vi "GetSetTempDir.vi"(3 "Path":refnum<vi>) -> ()   [LabVIEW 2009]
panel:
  out "rebinning after":dbl
  out "rebinning before":dbl
  in  "rebinning":dbl
  in  "false color palette":T1 {"Numeric 12" format="%.0x"; "Numeric 11" format="%.0x"; "Numeric 10" format="%.0x"; "Numeric 9" format="%.0x"; "Numeric 8" format="%.0x"; "Numeric 7" format="%.0x"; "Numeric 6" format="%.0x"; "Numeric 5" format="%.0x"; "Numeric 4" format="%.0x"; "Numeric 3" format="%.0x"; "Numeric 2" format="%.0x"; "Numeric" format="%.0x"}
  out "colors":u32[](array[colorbox])
  in  "ADC-Resolution":u16(ring) items=["8bit", "12bit", "4bit"]
  in  "raw data screen":bool
  in  "Fileformat":enum16{"Herty", "Ken", "SPC130", "HydraHarp"}(ring)
  in  "stop":bool
  in  "Path for .tmp-files":path
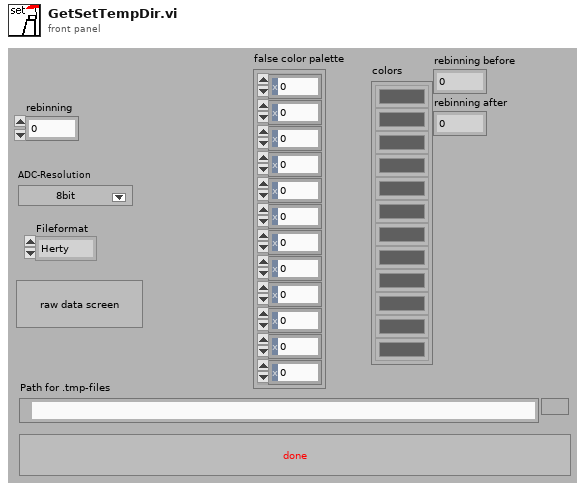
[diagram p1: front panel]
types:
  T1 = cluster{"Numeric":u32, "Numeric 2":u32, "Numeric 3":u32, "Numeric 4":u32, "Numeric 5":u32, "Numeric 6":u32, "Numeric 7":u32, "Numeric 8":u32, "Numeric 9":u32, "Numeric 10":u32, "Numeric 11":u32, "Numeric 12":u32}
  T2 = typedef "Settings.ctl" = cluster{"threshold":cluster{"max":u32, "min":u32}, "RGB or false color":bool, "16bit":bool, "log/lin axis":u16, "spotsize button":bool, "Pixelsize":u16, "autoscale x":bool, "autoscale y":bool, "correlation":bool, "ADC-Resolution":i32, "F2-lifetime":cluster{"display tau":bool, "display F2":bool, "Palette Number lifetime":enum32{"Gray", "Binary", "Gradient", "Rainbow", "Temperature"}, "Palette Number F2":enum32{"Gray", "Binary", "Gradient", "Rainbow", "Temperature"}, "max tau-Value":dbl, "min tau-Value":dbl, "max F2-Value":dbl, "min F2-Value":dbl}, "TAC-Window 1":u16, "TAC-Window 2":u16, "false color palette":cluster{"1":u32, "2":u32, "3":u32, "4":u32, "5":u32, "6":u32, "7":u32, "8":u32, "8 2":u32, "8 3":u32, "8 4":u32, "8 5":u32}, "rebinning":dbl}
  T3 = cluster{"1":u32, "2":u32, "3":u32, "4":u32, "5":u32, "6":u32, "7":u32, "8":u32, "8 2":u32, "8 3":u32, "8 4":u32, "8 5":u32}
  T4 = typedef "FIFOSettings_BH.ctt" = cluster{"Measurement":cluster{"Binning (ms)":sgl, "External Trigger Condition":u16, "Stop Condition:":u16, "Stop Count":dbl, "Buffer Size (Photons)":u16, "No of Channels":u16, "Ext Latch Delay":i16}, "ADC":cluster{"Module":u16, "ADC Resolution":i32, "Dither Range":i16, "Count Increment":i16, "Macro Time Clock":i16}, "SYNC":cluster{"SYNC ZC Level (mV)":sgl, "SYNC Freq Divider":i16, "SYNC Holdoff (ns)":sgl, "SYNC Threshold (mV)":sgl}, "TAC":cluster{"TAC Range (ns)":sgl, "TAC Gain":i16, "TAC Offset (%)":sgl, "TAC Limit Low (%)":sgl, "TAC Limit High (%)":sgl}, "CFD":cluster{"CFD Limit Low (mV)":sgl, "CFD Limit High (mV)":sgl, "CFD ZC Level (mV)":sgl, "CFD Holdoff (ns)":sgl}}
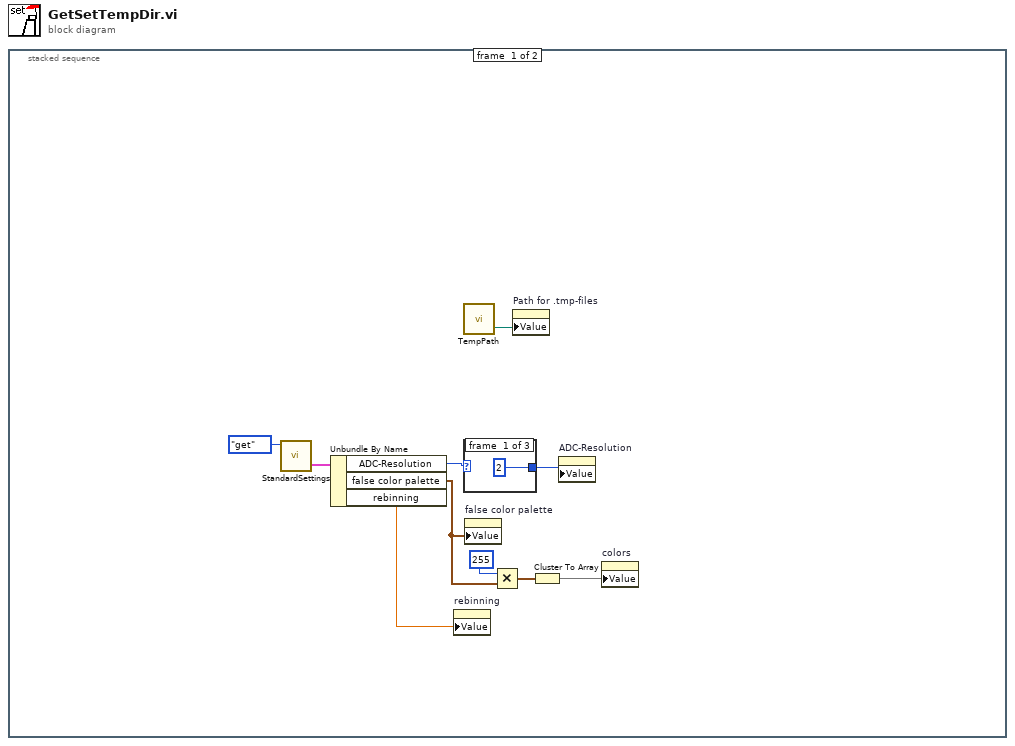
[diagram p0: block diagram]
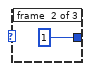
[diagram p2: hidden frame]
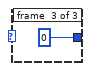
[diagram p3: hidden frame]
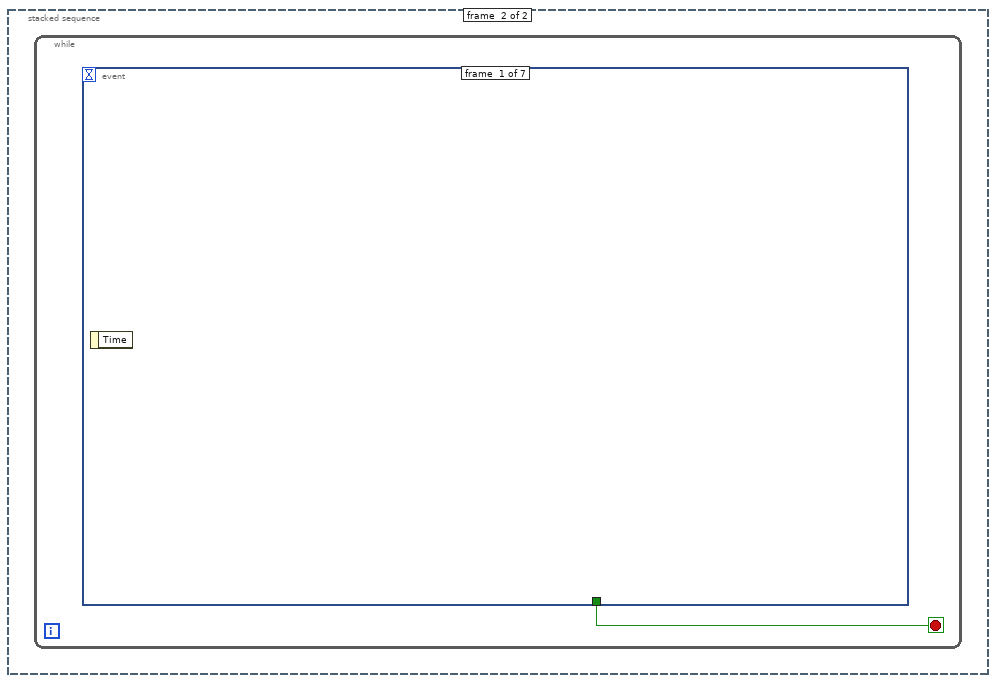
[diagram p4: hidden frame]
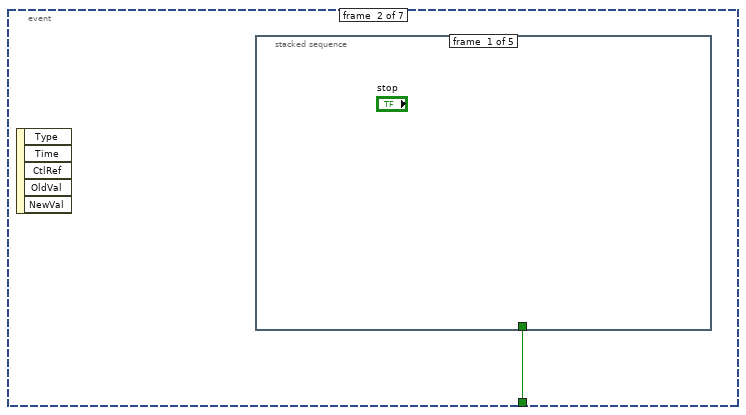
[diagram p5: hidden frame]
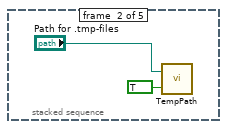
[diagram p6: hidden frame]
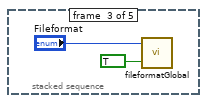
[diagram p7: hidden frame]
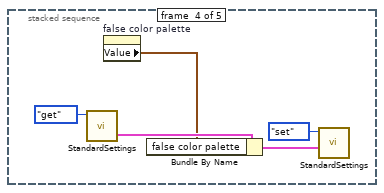
[diagram p8: hidden frame]
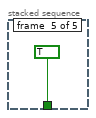
[diagram p9: hidden frame]
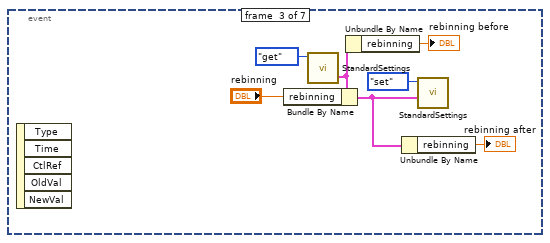
[diagram p10: hidden frame]
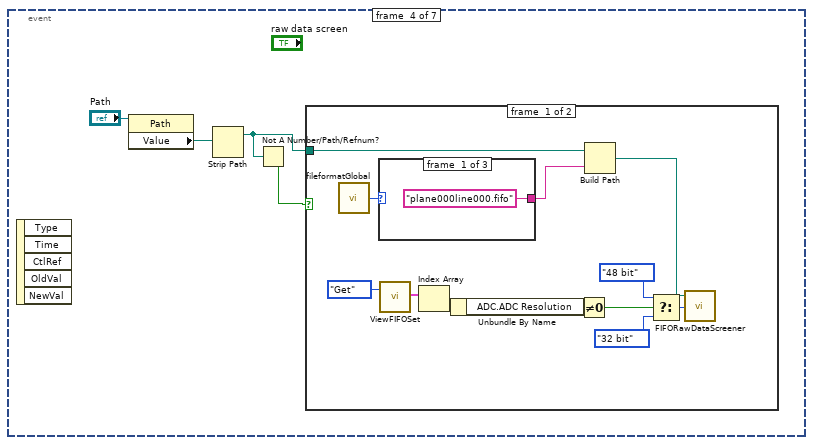
[diagram p11: hidden frame]
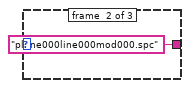
[diagram p12: hidden frame]
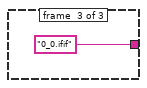
[diagram p13: hidden frame]
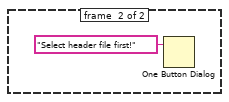
[diagram p14: hidden frame]
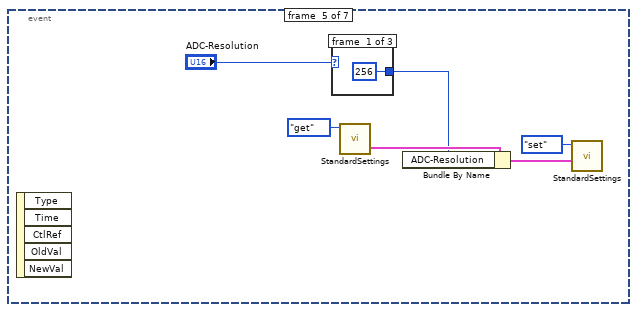
[diagram p15: hidden frame]
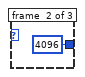
[diagram p16: hidden frame]
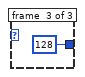
[diagram p17: hidden frame]
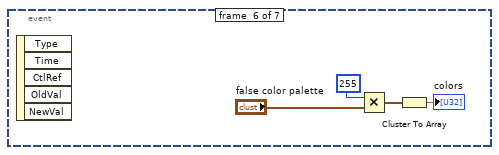
[diagram p18: hidden frame]
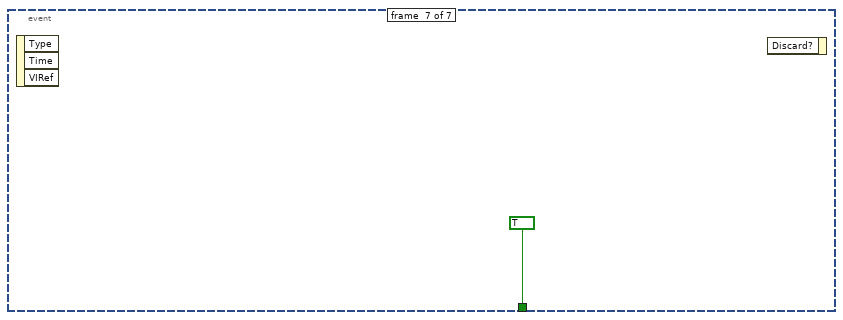
[diagram p19: hidden frame]
diagram:
  n1 = stacked-sequence {
    frame #0 {
      n2 = call "StandardSettings.vi"("Enum"=enum16{"Load", "get", "Save", "set"}."get") -> ("StandardSettings"=w8:T2)  [unwired: 4 in]
      n3 = Unbundle By Name(w8) -> ("ADC-Resolution"=w7:i32, "false color palette"=w2:T3, "rebinning"=w1:dbl)
      n4 = property on="rebinning" class="DigNum (strict)"("Value"=w1) -> ()  [unwired: 2 in, 2 out]
      n5 = call "TempPath.vi"() -> ("stripped path 2"=w10:path)  [unwired: 3 in]
      n6 = case shown="4096" w7 {
        tunnel: [u16 2 u16 1 u16 0] -> w6
        frame #0 {
        }
        frame #1 {
        }
        frame #2 {
        }
      }
      n7 = property on="false color palette" class="Clust (strict)"("Value"=w2) -> ()  [unwired: 2 in, 2 out]
      n8 = Multiply(x=u32 255, y=w2) -> (x*y=w3:T3)
      n9 = property on="Path for .tmp-files" class="Path"("Value"=w10) -> ()  [unwired: 2 in, 2 out]
      n10 = Cluster To Array(cluster=w3) -> (array=w5:u32[])
      n11 = property on="ADC-Resolution" class="Ring (strict)"("Value"=w6) -> ()  [unwired: 2 in, 2 out]
      n12 = property on="colors" class="Array (strict)"("Value"=w5) -> ()  [unwired: 2 in, 2 out]
    }
    frame #1 {
      n13 = while {
        stop <- w14 stop-if-true
        n14 = event shown="[2] \"rebinning\": Value Change" {
          selector: _ -> [_ _ _ _ _ _ _]
          dyn-events: _ -> [_ _ _ _ _ _ _]
          timeout: _ -> [_ _ _ _ _ _ _]
          tunnel: [_ w15 _ _ _ _ TRUE] -> w14
          event #0 {
            n15 = event-data() -> ()  [unwired: 1 in, 1 out]
          }
          event #1 {
            n16 = event-data() -> ()  [unwired: 1 in, 5 out]
            n17 = stacked-sequence {
              tunnel: [_ _ _ _ TRUE] -> w15
              frame #0 {
              }
              frame #1 {
                n18 = call "TempPath.vi"("change"=TRUE, "stripped path"="Path for .tmp-files") -> ()  [unwired: 1 in, 1 out]
              }
              frame #2 {
                n19 = call "fileformatGlobal.vi"("changed"=TRUE, "Fileformat"="Fileformat") -> ()  [unwired: 1 out]
              }
              frame #3 {
                n20 = call "StandardSettings.vi"("Enum"=enum16{"Load", "get", "Save", "set"}."get") -> ("StandardSettings"=w22:T2)  [unwired: 4 in]
                n21 = property on="false color palette" class="Clust (strict)"() -> ("Value"=w20:T1)  [unwired: 2 in, 2 out]
                n22 = Bundle By Name(cluster=w22, "false color palette"=w20) -> (w21:T2)
                n23 = call "StandardSettings.vi"("StandardSettings"=w21, "Enum"=enum16{"Load", "get", "Save", "set"}."set") -> ()  [unwired: 3 in, 1 out]
              }
              frame #4 {
              }
            }
          }
          event #2 {
            n24 = event-data() -> ()  [unwired: 1 in, 5 out]
            n25 = call "StandardSettings.vi"("Enum"=enum16{"Load", "get", "Save", "set"}."get") -> ("StandardSettings"=w29:T2)  [unwired: 4 in]
            n26 = Bundle By Name(cluster=w29, "rebinning"="rebinning") -> (w28:T2)
            n27 = Unbundle By Name(w29) -> ("rebinning"=→"rebinning before":dbl)
            n28 = Unbundle By Name(w28) -> ("rebinning"=→"rebinning after":dbl)
            n29 = call "StandardSettings.vi"("StandardSettings"=w28, "Enum"=enum16{"Load", "get", "Save", "set"}."set") -> ()  [unwired: 3 in, 1 out]
          }
          event #3 {
            n30 = event-data() -> ()  [unwired: 1 in, 5 out]
            n31 = property class="Path"(reference="Path") -> ("Value"=w36:path)  [unwired: 1 in, 2 out]
            n32 = Strip Path(path=w36) -> (stripped path=w35:path)  [unwired: 1 out]
            n33 = Not A Number/Path/Refnum?(number/path/refnum=w35) -> (NaN/Path/Refnum?=w34:bool)
            n34 = case shown="False" w34 {
              tunnel: w35 -> [w39 _]
              frame #0 {
                n35 = call "fileformatGlobal.vi"() -> ("fileformat out"=w41:enum16{"Herty", "Ken", "SPC130", "HydraHarp"})  [unwired: 2 in]
                n36 = case shown="\"SPC130\"" w41 {
                  tunnel: ["plane000line000.fifo" ("name or relative path") "plane000line000mod000.spc" ("name or relative path") "0_0.ifif" ("name or relative path")] -> w40
                  frame #0 {
                  }
                  frame #1 {
                  }
                  frame #2 {
                  }
                }
                n37 = call "ViewFIFOSet.vi"("Enum"=enum16{"Display", "change", "Get", "Set"}."Get") -> ("FIFO Settings (Array)"=w47:T4[])  [unwired: 1 in]
                n38 = Index Array(array=w47) -> (element=w37:T4)  [unwired: 1 in]
                n39 = Unbundle By Name(w37) -> ("ADC.ADC Resolution"=w43:i32)
                n40 = Not Equal To 0?(x=w43) -> (x != 0?=w42:bool)
                n41 = Build Path(base path=w39, name or relative path=w40) -> (appended path=w38:path)
                n42 = Select(t=enum16{"32 bit", "48 bit"}."48 bit" ("File Type"), s=w42, f=enum16{"32 bit", "48 bit"}."32 bit" ("File Type")) -> (s? t:f=w46:enum16{"32 bit", "48 bit"})
                n43 = call "FIFORawDataScreener.vi"("File Type"=w46, "Path"=w38) -> ()  [unwired: 2 in]
              }
              frame #1 {
                n44 = One Button Dialog(message="Select header file first!") -> ()  [unwired: 1 in, 1 out]
              }
            }
          }
          event #4 {
            n45 = event-data() -> ()  [unwired: 1 in, 5 out]
            n46 = case shown="1" "ADC-Resolution" {
              tunnel: [256 4096 128] -> w53
              frame #0 {
              }
              frame #1 {
              }
              frame #2 {
              }
            }
            n47 = call "StandardSettings.vi"("Enum"=enum16{"Load", "get", "Save", "set"}."get") -> ("StandardSettings"=w56:T2)  [unwired: 4 in]
            n48 = Bundle By Name(cluster=w56, "ADC-Resolution"=w53) -> (w57:T2)
            n49 = call "StandardSettings.vi"("StandardSettings"=w57, "Enum"=enum16{"Load", "get", "Save", "set"}."set") -> ()  [unwired: 3 in, 1 out]
          }
          event #5 {
            n50 = event-data() -> ()  [unwired: 1 in, 5 out]
            n51 = Multiply(x=u32 255, y="false color palette") -> (x*y=w64:T1)
            n52 = Cluster To Array(cluster=w64) -> (array=→"colors":u32[])
          }
          event #6 {
            n53 = event-data() -> ()  [unwired: 1 in, 3 out]
            n54 = event-data() -> ()  [unwired: 2 in, 1 out]
          }
        }
      }
    }
  }
